vi "readSignalFile_NIRS.vi"(2 "Путь к записи сигнала":path=path "C:/Users/ira_1/OneDrive/Рабочий стол/samples.bin", 3 "Целое число строк записанного файла":i32=50) -> (1 "Array 2":cdb[][](array[numeric]))   [LabVIEW 2020]
panel:
  out "size(s)":i32[](array[numeric])
  out "Array":dbl[][](array[numeric])
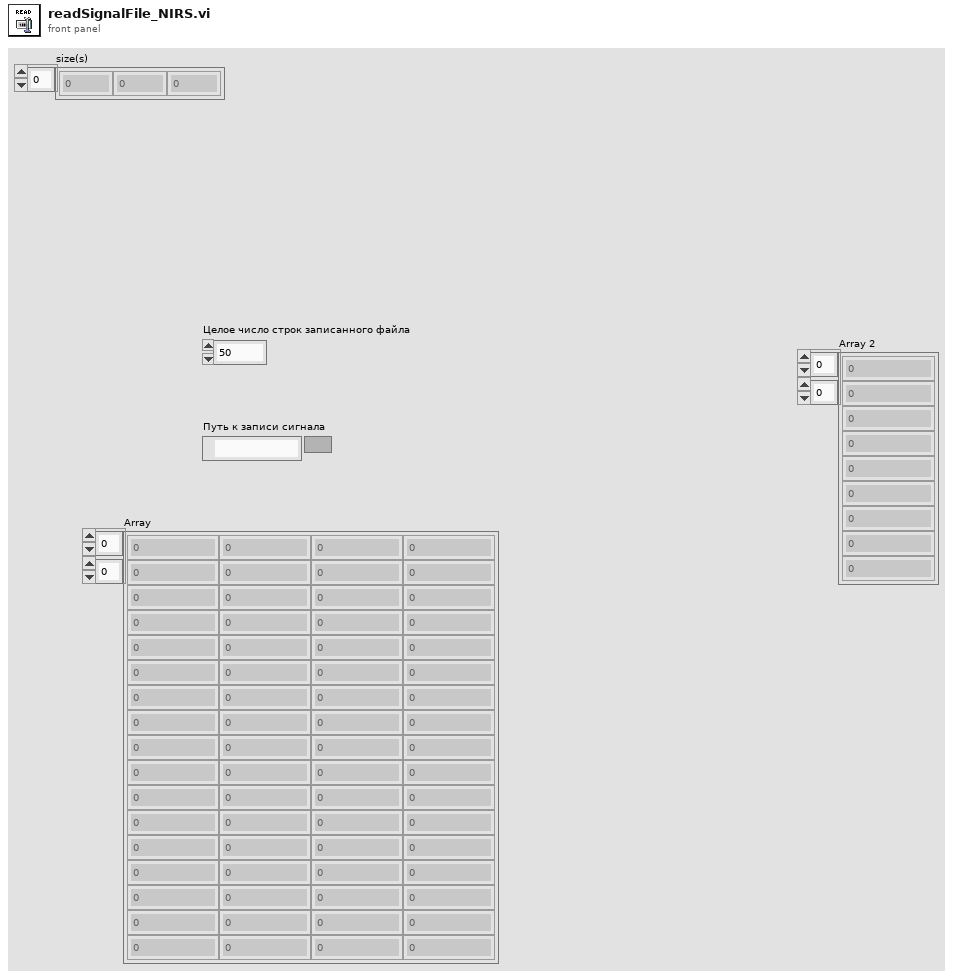
[diagram p1: front panel]
types:
  T1 = enum16{"open", "replace", "create", "open or create", "replace or create", "replace or create with confirmation"}
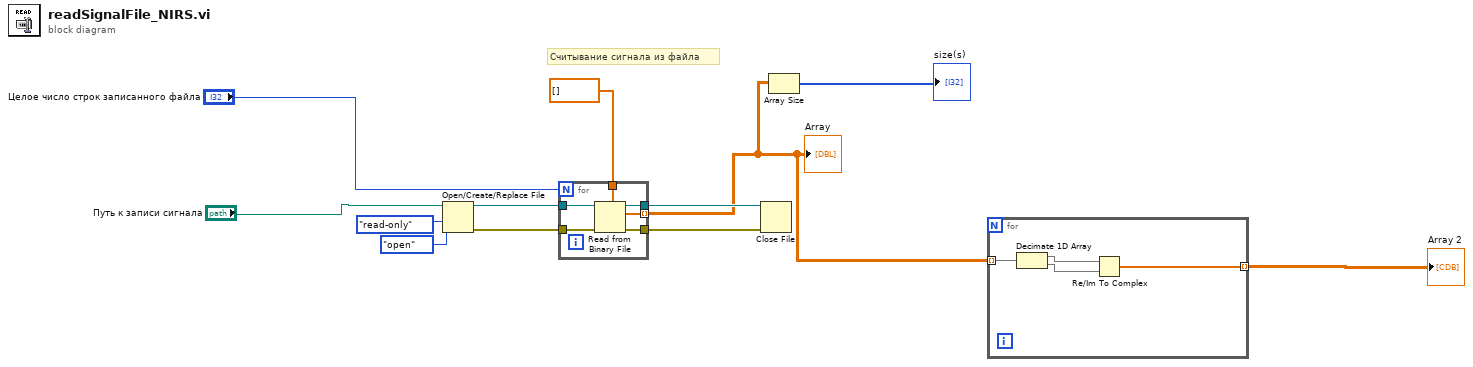
[diagram p0: block diagram]
diagram:
  # "Считывание сигнала из файла"
  n1 = Open/Create/Replace File(file path (use dialog)="Путь к записи сигнала", operation (0:open)=T1."open", access (0:read/write)=enum16{"read/write", "read-only", "write-only"}."read-only") -> (refnum out=w12:refnum<file>, error out=w11:errorcluster)  [unwired: 3 in, 1 out]
  n2 = for {
    N: "Целое число строк записанного файла" -> [_]
    tunnel: w12 -> [w18]
    tunnel: w11 -> [w17]
    tunnel: dbl[] [] -> [w16]
    tunnel: [w15] -> w3 mode=indexing
    tunnel: [w14] -> w7
    tunnel: [w13] -> w6
    n3 = Read from Binary File(5:w16, 8:w17, 11:w18) -> (0:w13:errorcluster, 2:w15:dbl[], 3:w14:refnum<file>)  [unwired: 3 in, 1 out]
  }
  "Array" <- w3
  n4 = Close File(refnum=w7, error in=w6) -> ()  [unwired: 2 out]
  n5 = Array Size(array=w3) -> (size(s)=→"size(s)":i32[])
  n6 = for {
    tunnel: w3 -> [w22] mode=indexing
    tunnel: [w19] -> w1 mode=indexing
    n7 = Decimate 1D Array(w22) -> (w21:dbl[], w20:dbl[])
    n8 = Re/Im To Complex(1:w20, 2:w21) -> (0:w19:cdb[])
  }
  "Array 2" <- w1
